vi "Com2Visa.vi"(11 "Portnumber":i32) -> (3 "VISA Refnum out":refnum<visa-resource-name>)   [LabVIEW 2017]
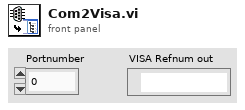
[diagram p1: front panel]
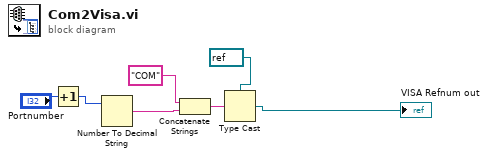
[diagram p0: block diagram]
diagram:
  n1 = Increment(x="Portnumber") -> (x+1=w5:i32)
  n2 = Number To Decimal String(number=w5) -> (decimal integer string=w6:string)  [unwired: 1 in]
  n3 = Concatenate Strings("COM" ("string"), w6) -> (w1:string)
  n4 = Type Cast(type=refnum<visa-resource-name> refnum, x=w1) -> (*(type *) &x=→"VISA Refnum out":refnum<visa-resource-name>)
